vi "GetTimeStampForMsg.vi"(8 "error in (no error)":errorcluster, 10 "SpyMessage{}":T1={"StatusBitField"=0, "StatusBitField2"=0, "TimeHardware"=0, "TimeHardware2"=0, "TimeSystem"=0, "TimeSystem2"=0, "TimeStampHardwareID"=0, "TimeStampHardwareID2"=0, "NetworkID"=0, "NodeID"=0, "Protocol"=0, "MessagePieceID"=0, "ColorID"=0, "NumberBytesHeader"=0, "NumberBytesData"=0, "DescriptionID"=0, "ArbIDOrHeader"=0, "Data [8]"=[0, 0, 0, 0, 0, 0, 0, 0], "AckBytes [8]"=[0, 0, 0, 0, 0, 0, 0, 0], "Value"=0.0, "MiscData"=0} {"AckBytes [8]" format="%.0x"; "Data [8]" format="%.0x"; "ArbIDOrHeader" format="%.0x"; "DescriptionID" format="%.0x"; "NetworkID" format="%.0x"}, 11 "hObject":i32) -> (0 "error out":errorcluster, 1 "pTimeStamp":dbl, 3 "hObject Out":i32)   [LabVIEW 2018]
doc: "this vi returns the timestamp of the input message\n\n12/21/2010 1.0.0 jyg\n- initial release"
uses:
  ctl spymessage.ctl
  icsneo40.dll
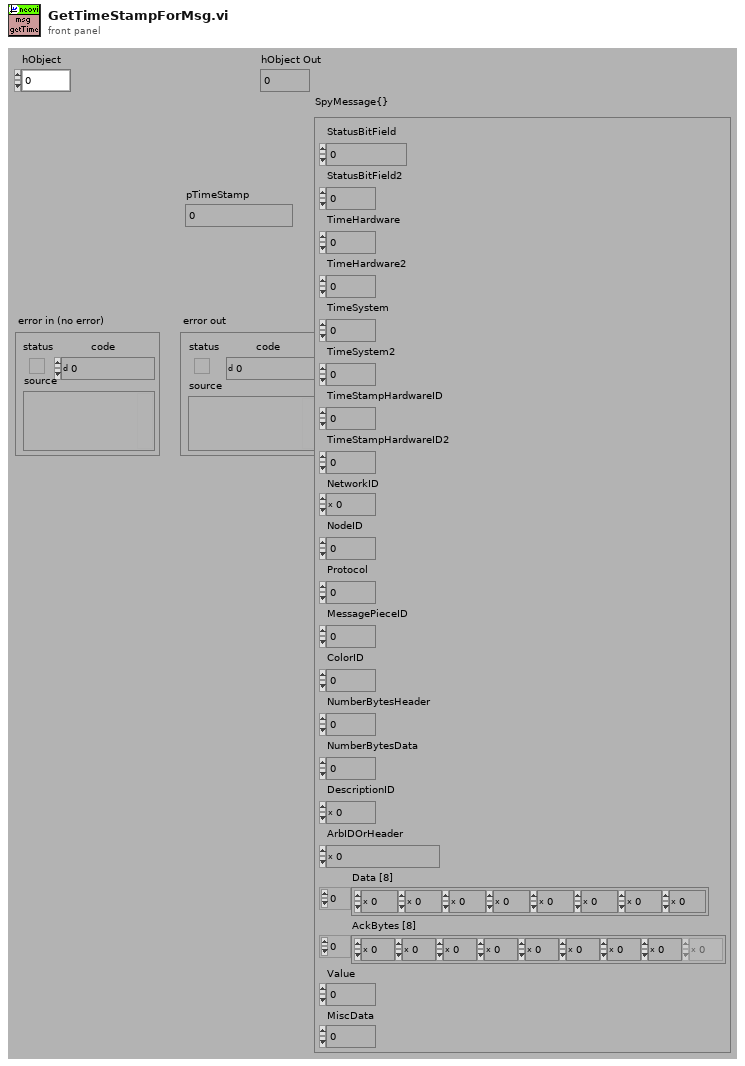
[diagram p1: front panel]
types:
  T1 = typedef "ctl spymessage.ctl" = cluster{"StatusBitField":u32, "StatusBitField2":u32, "TimeHardware":u32, "TimeHardware2":u32, "TimeSystem":u32, "TimeSystem2":u32, "TimeStampHardwareID":u8, "TimeStampHardwareID2":u8, "NetworkID":u8, "NodeID":u8, "Protocol":u8, "MessagePieceID":u8, "ColorID":u8, "NumberBytesHeader":u8, "NumberBytesData":u8, "DescriptionID":u16, "ArbIDOrHeader":u32, "Data [8]":u8[], "AckBytes [8]":u8[], "Value":sgl, "MiscData":u8}
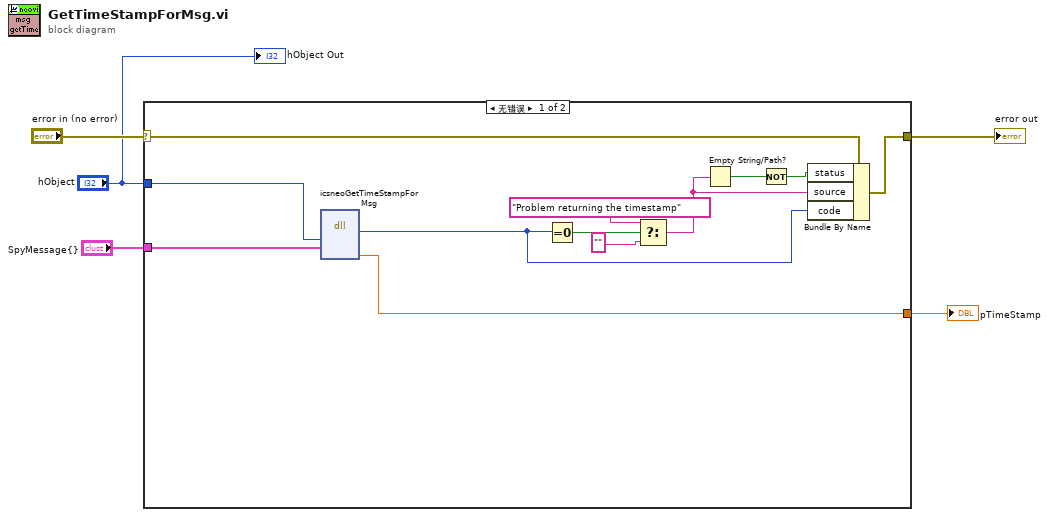
[diagram p0: block diagram]
diagram:
  n1 = case shown="无错误" "error in (no error)" {
    selector: "error in (no error)" -> [w13 w18]
    tunnel: "hObject" -> [w8 _]
    tunnel: [w14 w18] -> w5
    tunnel: [w7 _] -> w2
    tunnel: "SpyMessage{}" -> [w6 _]
    frame No Error {
      n2 = dll-call lib="icsneo40.dll" fn="icsneoGetTimeStampForMsg"("hObject"=w8, "pMsg"=w6) -> ("return type"=w12:i32, "pNumberOfMessages"=w7:dbl)  [unwired: 5 in, 3 out]
      n3 = Equal To 0?(x=w12) -> (x = 0?=w11:bool)
      n4 = Select(t="Problem returning the timestamp", s=w11, f="") -> (s? t:f=w10:string)
      n5 = Empty String/Path?(string/path=w10) -> (empty?=w16:bool)
      n6 = Not(x=w16) -> (.not. x?=w15:bool)
      n7 = Bundle By Name(cluster=w13, "status"=w15, "source"=w10, "code"=w12) -> (w14:errorcluster)
    }
    frame Error {
    }
  }
  "error out" <- w5
  "pTimeStamp" <- w2
  "hObject Out" <- "hObject"
